vi "4_5 Construct a VI Pro1.vi"() -> ()   [LabVIEW 2025]
panel:
  in  "stop":bool
  out "Y = 0":bool
  out "?":dbl
  out "Y - X":dbl
  in  "Y":dbl
  in  "X":dbl
  # "X / Y"
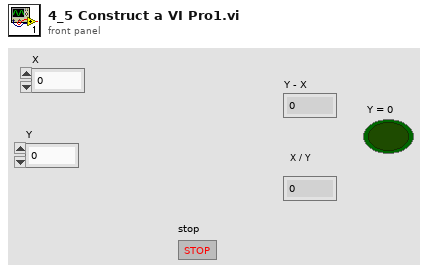
[diagram p1: front panel]
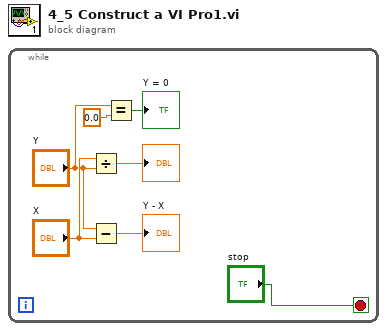
[diagram p0: block diagram]
diagram:
  n1 = while {
    stop <- "stop" stop-if-true
    n2 = Divide(x="X", y="Y") -> (x/y=→"?":dbl)
    n3 = Subtract(x="Y", y="X") -> (x-y=→"Y - X":dbl)
    n4 = Equal?(x="Y", y=0.0) -> (x = y?=→"Y = 0":bool)
  }
